vi "Actor Core.vi"(8 "error in":errorcluster, 11 "BASE.Device in":refnum<class "BASE.Device.lvclass">) -> (0 "error out":errorcluster, 3 "Actor out":refnum<class "Actor.lvclass">)   [LabVIEW 2019, in "BASE.Device.lvlib" / "BASE.Device.lvclass"]
doc: "(<B>Filename</B>: Actor Framework.lvlib:Actor.lvclass:Actor Core.vi)\n\nReceives messages to the actor, reacts to them, and initiates any error handling that may shut the actor down.\n\nDescendant classes may override this VI to append parallel tasks for the actor to complete while it handles messages. Overrides use the Call Parent Method node."
uses:
  BASE.Device.lvclass
  <vilib>/ActorFramework/Actor/Actor.lvclass
  config--cluster.ctl
  BASE.Device.lvclass/BASE.Device.ctl
  BASE/BASE/BASE.lvclass
panel:
  out "config":T1
  out "Run Read State":bool
  out "Run Disconnect":bool
  out "Run Check Connection":bool
  out "Run Connect":bool
  out "Connected?":bool
  in  "Stop":bool
  # "===Actor Core Status==="
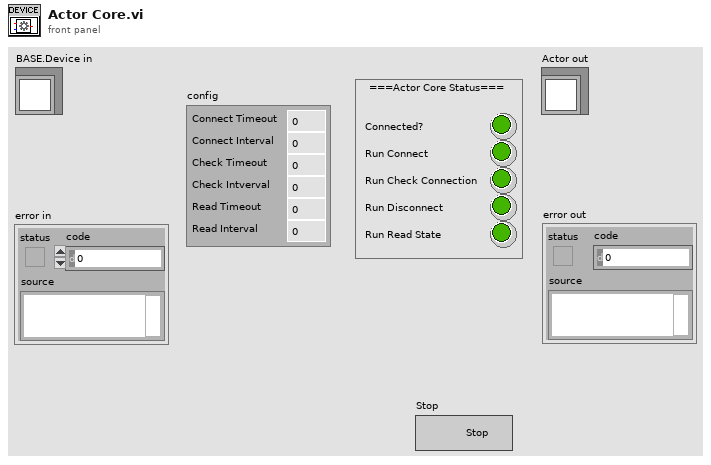
[diagram p1: front panel]
types:
  T1 = typedef "BASE.Device.lvlib/BASE.Device.lvclass/config--cluster.ctl" = cluster{"Connect Timeout":i32, "Connect Interval":u32, "Check Timeout":i32, "Check Intverval":u32, "Read Timeout":i32, "Read Interval":u32}
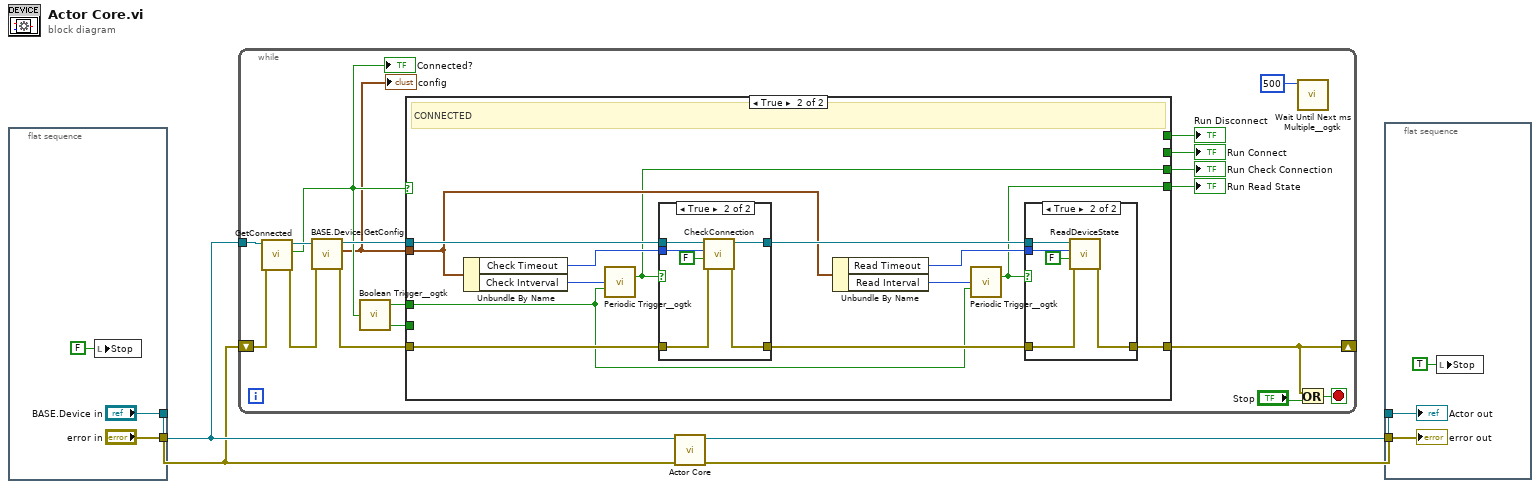
[diagram p0: block diagram]
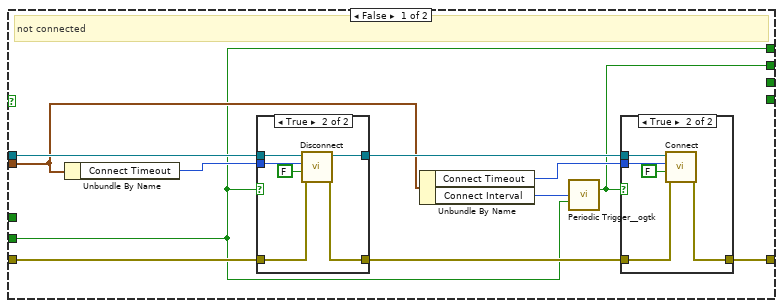
[diagram p2: hidden frame]
diagram:
  n1 = flat-sequence {
    tunnel: ["BASE.Device in"] -> w2
    tunnel: ["error in"] -> w1
    frame #0 {
      n2 = local write "Stop"(FALSE ("Stop")) -> ()
    }
  }
  n3 = while {
    tunnel: w2 -> [w20]
    shift-right: [w25] -> _
    shift-left: w1 -> [w18]
    stop <- w23 stop-if-true
    n4 = call "GetConnected.vi"("error in (no error)"=w18, "BASE.Device in"=w20) -> ("error out"=w15:errorcluster, "Connected?"=w16:bool, "BASE.Device out"=w19:refnum<class "BASE.Device.lvclass">)  [unwired: 7 in]
    "Connected?" <- w16
    n5 = call "BASE.Device.GetConfig.vi"("error in (no error)"=w15, "BASE.Device in"=w19) -> ("error out"=w14:errorcluster, "config"=w13:T1, "BASE.Device out"=w17:refnum<class "BASE.Device.lvclass">)  [unwired: 7 in]
    "config" <- w13
    n6 = call <userlib>:"Boolean Trigger__ogtk.vi"("Boolean Input"=w16) -> ("Rising Edge"=w21:bool, "Falling Edge"=w22:bool)  [unwired: 1 in]
    n7 = case shown="True" w16 {
      tunnel: w17 -> [w35 w61]
      tunnel: w14 -> [w34 w60]
      tunnel: [w30 w55] -> w25
      tunnel: w22 -> [w26 _]
      tunnel: w21 -> [_ w54]
      tunnel: w13 -> [w28 w53]
      tunnel: [_ w52] -> w12
      tunnel: [_ w51] -> w11
      tunnel: [w27 _] -> w10
      tunnel: [w26 _] -> w9
      frame False {
        # "not connected"
        n8 = Unbundle By Name(w28) -> ("Connect Timeout"=w36:i32)
        n9 = case shown="True" w26 {
          tunnel: [w44 w49] -> w32
          tunnel: w36 -> [_ w45]
          tunnel: w35 -> [w43 w47]
          tunnel: w34 -> [w44 w50]
          tunnel: [w43 w48] -> w31
          frame False {
          }
          frame True {
            n10 = call "Disconnect.vi"("error in (no error)"=w50, "Blocking?"=FALSE, "Timeout (5000 ms)"=w45, "BASE.Device in"=w47) -> ("error out"=w49:errorcluster, "BASE.Device out"=w48:refnum<class "BASE.Device.lvclass">)  [unwired: 6 in]
          }
        }
        n11 = Unbundle By Name(w28) -> ("Connect Timeout"=w33:i32, "Connect Interval"=w29:u32)
        n12 = call <userlib>:"Periodic Trigger__ogtk.vi"("time (ms)"=w29, "reset"=w26) -> ("Triggered"=w27:bool)  [unwired: 11 in, 2 out]
        n13 = case shown="True" w27 {
          tunnel: [w37 w41] -> w30
          tunnel: w33 -> [_ w38]
          tunnel: w31 -> [_ w40]
          tunnel: w32 -> [w37 w42]
          frame False {
          }
          frame True {
            n14 = call "Connect.vi"("error in (no error)"=w42, "Blocking?"=FALSE, "Timeout (5000 ms)"=w38, "BASE.Device in"=w40) -> ("error out"=w41:errorcluster)  [unwired: 6 in, 1 out]
          }
        }
      }
      frame True {
        # "CONNECTED"
        n15 = Unbundle By Name(w53) -> ("Check Timeout"=w62:i32, "Check Intverval"=w63:u32)
        n16 = call <userlib>:"Periodic Trigger__ogtk.vi"("time (ms)"=w63, "reset"=w54) -> ("Triggered"=w51:bool)  [unwired: 11 in, 2 out]
        n17 = case shown="True" w51 {
          tunnel: [w71 w73] -> w57
          tunnel: w62 -> [_ w76]
          tunnel: w61 -> [w70 w77]
          tunnel: w60 -> [w71 w74]
          tunnel: [w70 w72] -> w56
          frame False {
          }
          frame True {
            n18 = call "CheckConnection.vi"("error in (no error)"=w74, "Blocking?"=FALSE, "Timeout (5000 ms)"=w76, "BASE.Device in"=w77) -> ("error out"=w73:errorcluster, "BASE.Device out"=w72:refnum<class "BASE.Device.lvclass">)  [unwired: 6 in]
          }
        }
        n19 = Unbundle By Name(w53) -> ("Read Timeout"=w59:i32, "Read Interval"=w58:u32)
        n20 = call <userlib>:"Periodic Trigger__ogtk.vi"("time (ms)"=w58, "reset"=w54) -> ("Triggered"=w52:bool)  [unwired: 11 in, 2 out]
        n21 = case shown="True" w52 {
          tunnel: [w64 w68] -> w55
          tunnel: w59 -> [_ w65]
          tunnel: w56 -> [_ w69]
          tunnel: w57 -> [w64 w67]
          frame False {
          }
          frame True {
            n22 = call "ReadDeviceState.vi"("error in (no error)"=w67, "Blocking?"=FALSE, "Timeout (5000 ms)"=w65, "BASE.Device in"=w69) -> ("error out"=w68:errorcluster)  [unwired: 6 in, 1 out]
          }
        }
      }
    }
    "Run Read State" <- w12
    "Run Check Connection" <- w11
    "Run Connect" <- w10
    "Run Disconnect" <- w9
    n23 = call <userlib>:"Wait Until Next ms Multiple__ogtk.vi"("milliseconds to wait"=u32 500) -> ()  [unwired: 9 in, 2 out]
    n24 = Or(x=w25, y="Stop") -> (x .or. y?=w23:bool)
  }
  n25 = call-parent "Actor Core.vi"("error in"=w1, "Actor in"=w2) -> ("error out"=w4:errorcluster, "Actor out"=w3:refnum<class "Actor.lvclass">)  [unwired: 8 in]
  n26 = flat-sequence {
    tunnel: w4 -> [w80]
    tunnel: w3 -> [w79]
    frame #0 {
      n27 = local write "Stop"(TRUE ("Stop")) -> ()
      "error out" <- w80
      "Actor out" <- w79
    }
  }
